vi "16进制to2进制.vi"(1 "16进制字符串":string) -> (0 "2进制字符串":string)   [LabVIEW 2014]
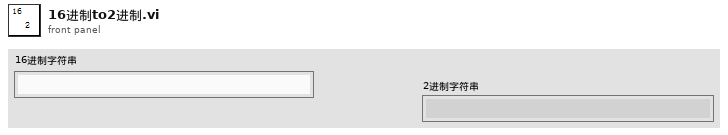
[diagram p1: front panel]
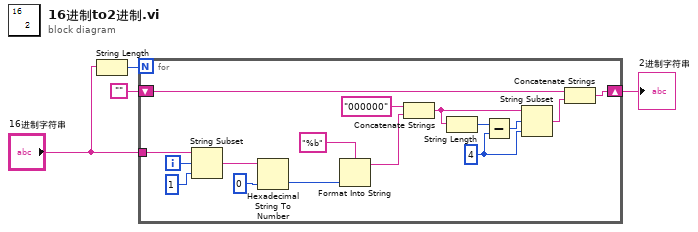
[diagram p0: block diagram]
diagram:
  n1 = String Length(string="16进制字符串") -> (length=w4:i32)
  n2 = for {
    N: w4 -> [_]
    tunnel: "16进制字符串" -> [w17]
    shift-right: [w5] -> w1
    shift-left: "" -> [w6]
    i -> [w16]
    w11 = u16 4 ("默认(0 U32)")
    n3 = String Subset(string=w17, offset (0)=w16, length (rest)=1 ("长度（剩余）")) -> (substring=w14:string)
    n4 = Hexadecimal String To Number(string=w14, default (0uL)=u8 0 ("默认(0 U32)")) -> (number=w18:u8)  [unwired: 1 in, 1 out]
    n5 = Format Into String(format string="%b" ("格式字符串"), w18) -> (resulting string=w13:string)  [unwired: 2 in, 1 out]
    n6 = Concatenate Strings("000000" ("字符串"), w13) -> (w8:string)
    n7 = String Length(string=w8) -> (length=w9:i32)
    n8 = Subtract(x=w9, y=w11) -> (x-y=w10:i32)
    n9 = String Subset(string=w8, offset (0)=w10, length (rest)=w11) -> (substring=w7:string)
    n10 = Concatenate Strings(w6, w7) -> (w5:string)
  }
  "2进制字符串" <- w1
